vi "Part Type to Stamp Type.vi"(8 "error in":errorcluster, 11 "Stamp Type":T1) -> (0 "error out":errorcluster, 3 "Part Type":T2)   [LabVIEW 2011]
uses:
  Config Manager Class/Type Definitions/Part Type.ctl
  Config Manager Class/Type Definitions/Stamp Type.ctl
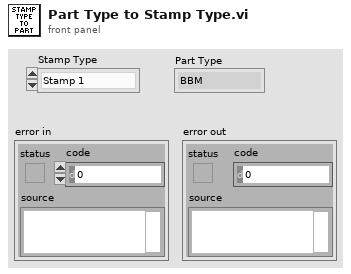
[diagram p1: front panel]
types:
  T1 = typedef "Stamp Type.ctl" = enum16{"Stamp 1", "Stamp 2", "Stamp 3", "Stamp 4", "Stamp 5"}
  T2 = typedef "Part Type.ctl" = enum16{"BBM", "HDI", "BARE HDI", "GLUERESERVOIR", "STAMP_1", "STAMP_2", "STAMP_3", "STAMP_4", "STAMP_5", "WEIGHT_1", "WEIGHT_2", "WEIGHT_3", "WEIGHT_4", "WEIGHT_5", "WEIGHT_6", "WEIGHT_7", "WEIGHT_8", "PICKER_TOOL", "GRABER_TOOL"}
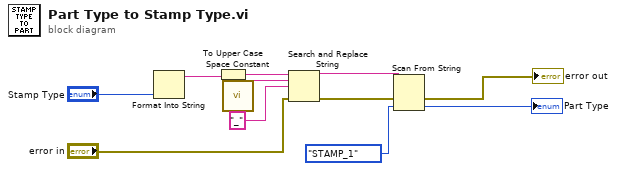
[diagram p0: block diagram]
diagram:
  n1 = Format Into String("Stamp Type") -> (resulting string=w11:string)  [unwired: 3 in, 1 out]
  n2 = To Upper Case(1:w11) -> (0:w10:string)
  n3 = call <vilib>:"Space Constant.vi"() -> ("String"=w9:string)
  n4 = Search and Replace String(input string=w10, search string=w9, replace string="_" ("replace string (\"\")"), error in="error in") -> (result string=w6:string, error out=w5:errorcluster)  [unwired: 4 in, 2 out]
  n5 = Scan From String(input string=w6, error in=w5, default 1=Part_Type."STAMP_1" ("Part Type")) -> (error out=→"error out":errorcluster, output 1=→"Part Type":T2)  [unwired: 2 in, 2 out]
